vi "CAN Uninitialize.vi"(8 "error in (no error)":errorcluster, 11 "Channel":u16) -> (0 "error out":errorcluster, 3 "function return":u32)   [LabVIEW 2025, in "PCAN2023.lvlib"]
doc: "Uninitializes one or all PCAN Channels initialized by CAN_Initialize\n\n\nTPCANStatus __stdcall CAN_Uninitialize(\n TPCANHandle Channel);"
uses:
  PCAN2023.lvlib
  PCANBasic.dll
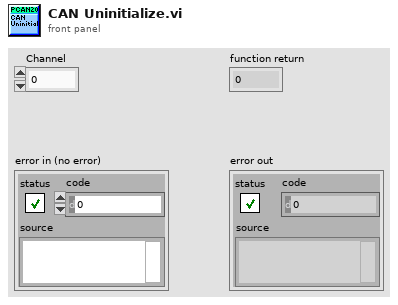
[diagram p1: front panel]
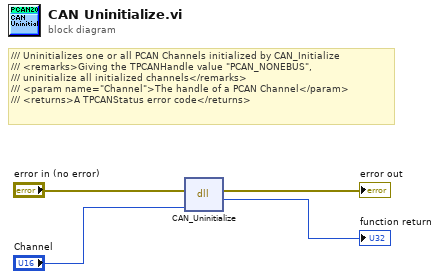
[diagram p0: block diagram]
diagram:
  # "/// Uninitializes one or all PCAN Channels initialized by CAN_Initialize\n/// <remarks>Giving the TPCANHandle value \"PCAN_NONEBUS\", \n/// uninitialize all initialized channels</remarks>\n/// <param name=\"Channel\">The handle of a PCAN Channel</param>\n/// <returns>A TPCANStatus error code</returns>"
  n1 = dll-call lib="PCANBasic.*" fn="CAN_Uninitialize"(error in="error in (no error)", "Channel"="Channel") -> (error out=→"error out":errorcluster, "return type"=→"function return":u32)  [unwired: 3 in, 1 out]
